vi "FGV Zustand Kalibrierung.vi"(6 "Aktionen":T2) -> (0 "Fehler":bool, 2 "Zustand Kalibrierung":T1)   [LabVIEW 2020, in "Auto Kalibrieren.lvlib"]
uses:
  Auto Kalibrieren.lvlib
  Aktionen FGV Zustand Kalibrierung.ctl
  Zustand Messgeraete Kalibrierung.ctl
  Stoerungen/Stoerungen Messgeraet/Aktionen Kommunikation Stoerung.ctl
  Stoerungen/Stoerungen.lvlib
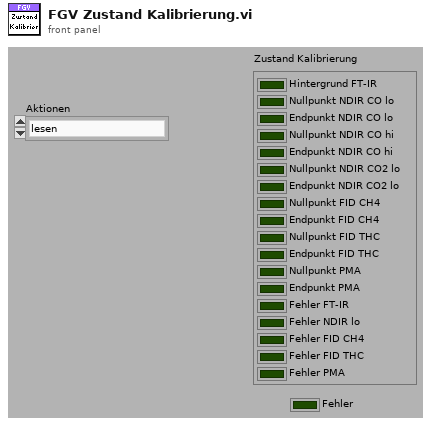
[diagram p1: front panel]
types:
  T1 = typedef "Auto Kalibrieren.lvlib/Zustand Messgeraete Kalibrierung.ctl" = cluster{"Hintergrund FT-IR":bool, "Nullpunkt NDIR CO lo":bool, "Endpunkt NDIR CO lo":bool, "Nullpunkt NDIR CO hi":bool, "Endpunkt NDIR CO hi":bool, "Nullpunkt NDIR CO2 lo":bool, "Endpunkt NDIR CO2 lo":bool, "Nullpunkt FID CH4":bool, "Endpunkt FID CH4":bool, "Nullpunkt FID THC":bool, "Endpunkt FID THC":bool, "Nullpunkt PMA":bool, "Endpunkt PMA":bool, "Fehler FT-IR":bool, "Fehler NDIR lo":bool, "Fehler FID CH4":bool, "Fehler FID THC":bool, "Fehler PMA":bool}
  T2 = typedef "Auto Kalibrieren.lvlib/Aktionen FGV Zustand Kalibrierung.ctl" = enum16{"lesen", "LÖSCHEN", "Hintergrund fertig", "Nullpunkt NDIR CO lo", "Endpunkt NDIR CO lo", "Nullpunkt NDIR CO hi", "Endpunkt NDIR CO hi", "Nullpunkt NDIR CO2 lo", "Endpunkt NDIR CO2 lo", "Nullpunkt FID CH4", "Endpunkt FID CH4", "Nullpunkt FID THC", "Endpunkt FID THC", "Nullpunkt PMA", "Endpunkt PMA", "Fehler FT-IR", "Fehler NDIR lo", "Fehler FID CH4", "Fehler FID THC", "Fehler PMA", "TIMEOUT"}
  T3 = typedef "Stoerungen.lvlib/Aktionen Kommunikation Stoerung.ctl" = enum16{"lesen", "init", "FT-IR Komm", "FT-IR Betriebsart", "FT-IR Hintergrund", "cRIO Komm", "PNS Komm", "Dichtheitstest", "Life Bit", "FTIR Komm AK", "PMA Komm", "FID Komm", "PMA Cal", "FID Ch4 Cal", "FID THC Cal", "Cal Timeout", "VFS 1 Komm", "VFS 2 Komm", "VFS 3 Komm", "VFS 4 Komm", "TRE 08 Komm", "CG-Test vorzeitig", "CG-Test Span 1", "CG-Test Span 2", "CG-Test Span 3", "CG-Test Messgas", "CG-Test löschen", "Test", "Amium AK", "AK Recept konfig", "AK Name konfig", "AK EKFG konfig"}
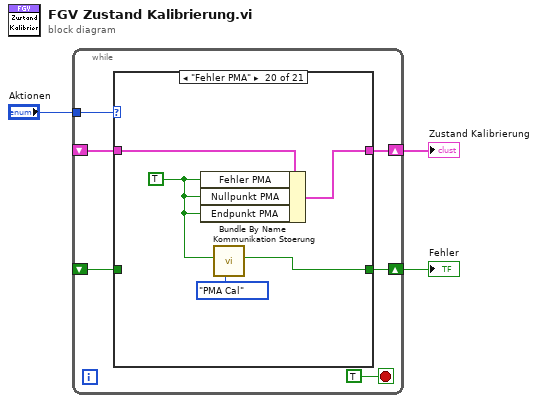
[diagram p0: block diagram]
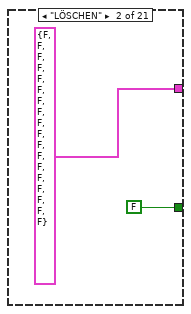
[diagram p3: hidden frame]
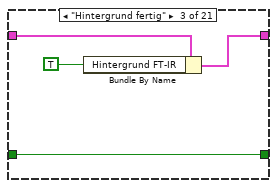
[diagram p4: hidden frame]
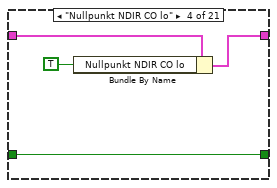
[diagram p5: hidden frame]
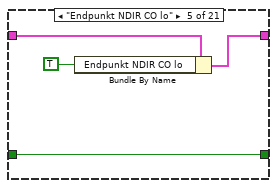
[diagram p6: hidden frame]
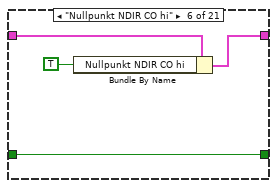
[diagram p7: hidden frame]
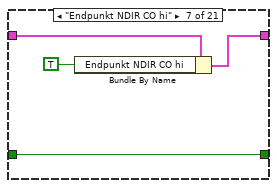
[diagram p8: hidden frame]
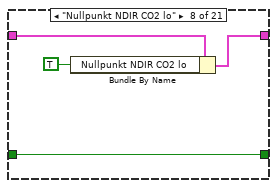
[diagram p9: hidden frame]
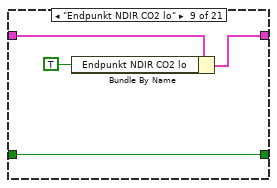
[diagram p10: hidden frame]
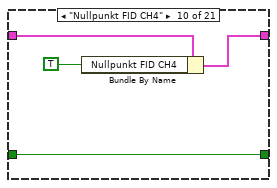
[diagram p11: hidden frame]
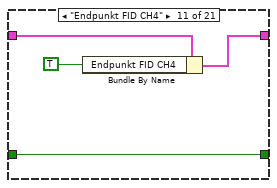
[diagram p12: hidden frame]
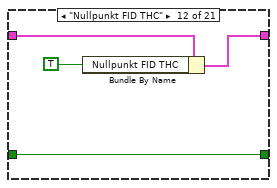
[diagram p13: hidden frame]
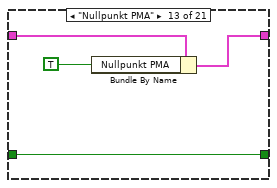
[diagram p14: hidden frame]
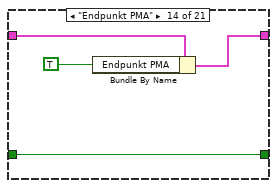
[diagram p15: hidden frame]
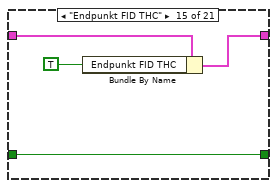
[diagram p16: hidden frame]
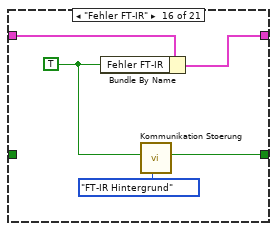
[diagram p17: hidden frame]
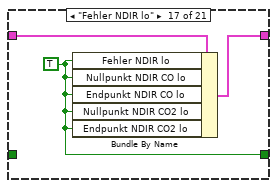
[diagram p18: hidden frame]
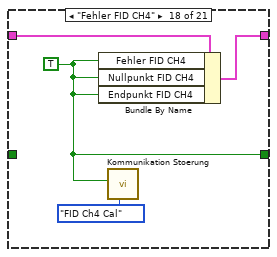
[diagram p19: hidden frame]
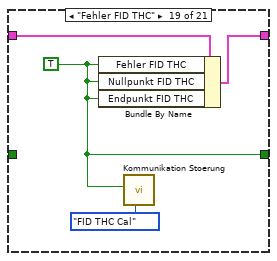
[diagram p20: hidden frame]
diagram:
  n1 = while {
    tunnel: "Aktionen" -> [w8]
    shift-right: [w7] -> w2
    shift-left: _ -> [w6]
    shift-right: [w5] -> w1
    shift-left: _ -> [w4]
    stop <- TRUE stop-if-true
    n2 = case shown="\"Fehler PMA\"" w8 {
      tunnel: [w11 T1 {"Hintergrund FT-IR"=FALSE, "Nullpunkt NDIR CO lo"=FALSE, "Endpunkt NDIR CO lo"=FALSE, "Nullpunkt NDIR CO hi"=FALSE, "Endpunkt NDIR CO hi"=FALSE, "Nullpunkt NDIR CO2 lo"=FALSE, "Endpunkt NDIR CO2 lo"=FALSE, "Nullpunkt FID CH4"=FALSE, "Endpunkt FID CH4"=FALSE, "Nullpunkt FID THC"=FALSE, "Endpunkt FID THC"=FALSE, "Nullpunkt PMA"=FALSE, "Endpunkt PMA"=FALSE, "Fehler FT-IR"=FALSE, "Fehler NDIR lo"=FALSE, "Fehler FID CH4"=FALSE, "Fehler FID THC"=FALSE, "Fehler PMA"=FALSE} ("Zustand Kalibrierung") w16 w20 w24 w28 w32 w36 w40 w44 w48 w52 w56 w60 w64 w68 w71 w75 w79 w83 w85] -> w7
      tunnel: w6 -> [w11 _ w17 w21 w25 w29 w33 w37 w41 w45 w49 w53 w57 w61 w65 w69 w72 w76 w80 w84 w85]
      tunnel: [w10 FALSE ("Hintergrund FT-IR") w14 w18 w22 w26 w30 w34 w38 w42 w46 w50 w54 w58 w62 w66 w70 w73 w77 w81 w86] -> w5
      tunnel: w4 -> [w10 _ w14 w18 w22 w26 w30 w34 w38 w42 w46 w50 w54 w58 w62 _ _ _ _ _ _]
      frame "lesen", Default {
      }
      frame "LÖSCHEN" {
      }
      frame "Hintergrund fertig" {
        n3 = Bundle By Name(cluster=w17, "Hintergrund FT-IR"=TRUE) -> (w16:T1)
      }
      frame "Nullpunkt NDIR CO lo" {
        n4 = Bundle By Name(cluster=w21, "Nullpunkt NDIR CO lo"=TRUE ("Hintergrund FT-IR")) -> (w20:T1)
      }
      frame "Endpunkt NDIR CO lo" {
        n5 = Bundle By Name(cluster=w25, "Endpunkt NDIR CO lo"=TRUE ("Hintergrund FT-IR")) -> (w24:T1)
      }
      frame "Nullpunkt NDIR CO hi" {
        n6 = Bundle By Name(cluster=w29, "Nullpunkt NDIR CO hi"=TRUE ("Hintergrund FT-IR")) -> (w28:T1)
      }
      frame "Endpunkt NDIR CO hi" {
        n7 = Bundle By Name(cluster=w33, "Endpunkt NDIR CO hi"=TRUE ("Hintergrund FT-IR")) -> (w32:T1)
      }
      frame "Nullpunkt NDIR CO2 lo" {
        n8 = Bundle By Name(cluster=w37, "Nullpunkt NDIR CO2 lo"=TRUE ("Hintergrund FT-IR")) -> (w36:T1)
      }
      frame "Endpunkt NDIR CO2 lo" {
        n9 = Bundle By Name(cluster=w41, "Endpunkt NDIR CO2 lo"=TRUE ("Hintergrund FT-IR")) -> (w40:T1)
      }
      frame "Nullpunkt FID CH4" {
        n10 = Bundle By Name(cluster=w45, "Nullpunkt FID CH4"=TRUE ("Hintergrund FT-IR")) -> (w44:T1)
      }
      frame "Endpunkt FID CH4" {
        n11 = Bundle By Name(cluster=w49, "Endpunkt FID CH4"=TRUE ("Hintergrund FT-IR")) -> (w48:T1)
      }
      frame "Nullpunkt FID THC" {
        n12 = Bundle By Name(cluster=w53, "Nullpunkt FID THC"=TRUE ("Hintergrund FT-IR")) -> (w52:T1)
      }
      frame "Nullpunkt PMA" {
        n13 = Bundle By Name(cluster=w57, "Nullpunkt PMA"=TRUE ("Hintergrund FT-IR")) -> (w56:T1)
      }
      frame "Endpunkt PMA" {
        n14 = Bundle By Name(cluster=w61, "Endpunkt PMA"=TRUE ("Hintergrund FT-IR")) -> (w60:T1)
      }
      frame "Endpunkt FID THC" {
        n15 = Bundle By Name(cluster=w65, "Endpunkt FID THC"=TRUE ("Hintergrund FT-IR")) -> (w64:T1)
      }
      frame "Fehler FT-IR" {
        w66 = TRUE ("Hintergrund FT-IR")
        n16 = Bundle By Name(cluster=w69, "Fehler FT-IR"=w66) -> (w68:T1)
        n17 = call "Kommunikation Stoerung.vi"("Aktionen"=Aktionen_Kommunikation_Stoerung."FT-IR Hintergrund", "ERROR"=w66) -> ()  [unwired: 9 in, 1 out]
      }
      frame "Fehler NDIR lo" {
        w70 = TRUE ("Hintergrund FT-IR")
        n18 = Bundle By Name(cluster=w72, "Fehler NDIR lo"=w70, "Nullpunkt NDIR CO lo"=w70, "Endpunkt NDIR CO lo"=w70, "Nullpunkt NDIR CO2 lo"=w70, "Endpunkt NDIR CO2 lo"=w70) -> (w71:T1)
      }
      frame "Fehler FID CH4" {
        w73 = TRUE ("Hintergrund FT-IR")
        n19 = Bundle By Name(cluster=w76, "Fehler FID CH4"=w73, "Nullpunkt FID CH4"=w73, "Endpunkt FID CH4"=w73) -> (w75:T1)
        n20 = call "Kommunikation Stoerung.vi"("Aktionen"=Aktionen_Kommunikation_Stoerung."FID Ch4 Cal", "ERROR"=w73) -> ()  [unwired: 9 in, 1 out]
      }
      frame "Fehler FID THC" {
        w77 = TRUE ("Hintergrund FT-IR")
        n21 = Bundle By Name(cluster=w80, "Fehler FID THC"=w77, "Nullpunkt FID THC"=w77, "Endpunkt FID THC"=w77) -> (w79:T1)
        n22 = call "Kommunikation Stoerung.vi"("Aktionen"=Aktionen_Kommunikation_Stoerung."FID THC Cal", "ERROR"=w77) -> ()  [unwired: 9 in, 1 out]
      }
      frame "Fehler PMA" {
        w81 = TRUE ("Hintergrund FT-IR")
        n23 = Bundle By Name(cluster=w84, "Fehler PMA"=w81, "Nullpunkt PMA"=w81, "Endpunkt PMA"=w81) -> (w83:T1)
        n24 = call "Kommunikation Stoerung.vi"("Aktionen"=Aktionen_Kommunikation_Stoerung."PMA Cal", "ERROR"=w81) -> ()  [unwired: 9 in, 1 out]
      }
      frame "TIMEOUT" {
        w86 = TRUE ("Hintergrund FT-IR")
        n25 = call "Kommunikation Stoerung.vi"("Aktionen"=Aktionen_Kommunikation_Stoerung."Cal Timeout", "ERROR"=w86) -> ()  [unwired: 9 in, 1 out]
      }
    }
  }
  "Zustand Kalibrierung" <- w2
  "Fehler" <- w1
